vi "initializeDefaultStyle.vi"(8 "error in (no error)":errorcluster, 11 "Heading in":refnum<class "Heading.lvclass">) -> (0 "error out":errorcluster, 3 "Heading out":refnum<class "Heading.lvclass">)   [LabVIEW 2020, in "Styles.lvlib" / "Heading.lvclass"]
uses:
  Heading.lvclass
  D:/Benjamin/Documents/Perso/Code/WC/LabVIEW_NPOI/src/Styles/Style/Style.lvclass
  Style/Style.lvclass
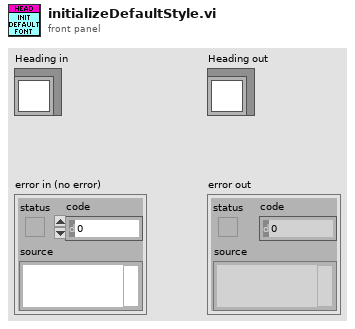
[diagram p1: front panel]
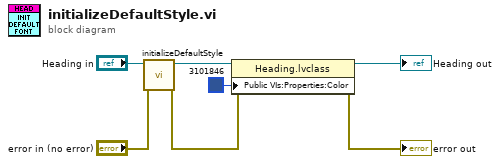
[diagram p0: block diagram]
diagram:
  n1 = call-parent "initializeDefaultStyle.vi"("error in (no error)"="error in (no error)", "Style in"="Heading in") -> ("error out"=w2:errorcluster, "Style out"=w7:refnum<class "Heading.lvclass">)  [unwired: 8 in]
  n2 = property class="Heading.lvclass"(reference=w7, error in=w2, "Public VIs:Properties:Color"=u32 3101846 ("Style:Color:Color")) -> (reference out=→"Heading out":refnum<class "Heading.lvclass">, error out=→"error out":errorcluster)
